vi "Median PtByPt.vi"(2 "initialize":bool, 3 "sample length":i32=100, 5 "x":dbl format="%0.2f") -> (0 "error":i32, 1 "median":dbl format="%0.2f")   [LabVIEW 2017, in "NI_PtbyPt.lvlib"]
doc: "Finds the median value of the set of input data points specified by <B>sample length</B> by sorting the values of the newest set of input data points and selecting the middle element(s) of the sorted set of data points."
uses:
  <vilib>/ptbypt/NI_PtbyPt.lvlib
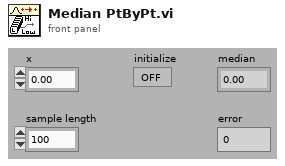
[diagram p1: front panel]
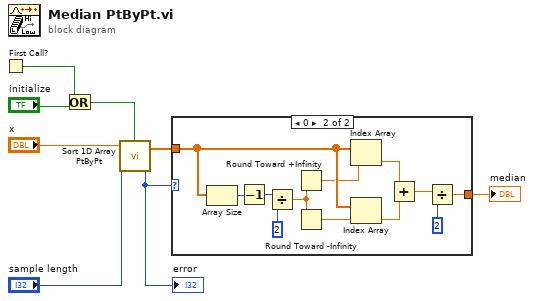
[diagram p0: block diagram]
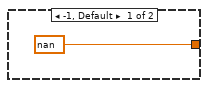
[diagram p2: hidden frame]
diagram:
  n1 = First Call?() -> (First Call?: T/F=w3:bool)
  n2 = Or(x=w3, y="initialize") -> (x .or. y?=w2:bool)
  n3 = call <vilib>:"Sort 1D Array PtByPt.vi"("initialize"=w2, "sample length"="sample length", "input data point"="x") -> ("error"=w1:i32, "sorted array"=w7:dbl[])  [unwired: 1 in]
  "error" <- w1
  n4 = case shown="0" w1 {
    tunnel: w7 -> [_ w18]
    tunnel: [nan w12] -> w6
    frame -1, Default {
    }
    frame 0 {
      n5 = Array Size(array=w18) -> (size(s)=w21:i32)
      n6 = Decrement(x=w21) -> (x-1=w19:i32)
      n7 = Divide(x=w19, y=2) -> (x/y=w11:dbl)
      n8 = Round Toward +Infinity(x=w11) -> (ceil(x): smallest int >= x=w10:dbl)
      n9 = Round Toward -Infinity(1:w11) -> (0:w17:dbl)
      n10 = Index Array(array=w18, index=w10) -> (element=w16:dbl)
      n11 = Index Array(array=w18, index=w17) -> (element=w15:dbl)
      n12 = Add(x=w16, y=w15) -> (x+y=w14:dbl)
      n13 = Divide(x=w14, y=2) -> (x/y=w12:dbl)
    }
  }
  "median" <- w6
